vi "Create Error Cluster Control.vi"(5 "Error Cluster Sink":refnum<vi>, 6 "relative position/next to refnum":T1, 8 "error in (no error)":errorcluster, 10 "Indicator ?":bool, 11 "Diagram":refnum<vi>) -> (0 "error out":errorcluster, 2 "Terminal":refnum<vi>, 3 "cluster ref":refnum<vi>)   [LabVIEW 2012, in "Scripting Tools.lvlib"]
uses:
  Scripting Tools.lvlib
  <vilib>/Utility/miscctls.llb/LVPointTypeDef.ctl
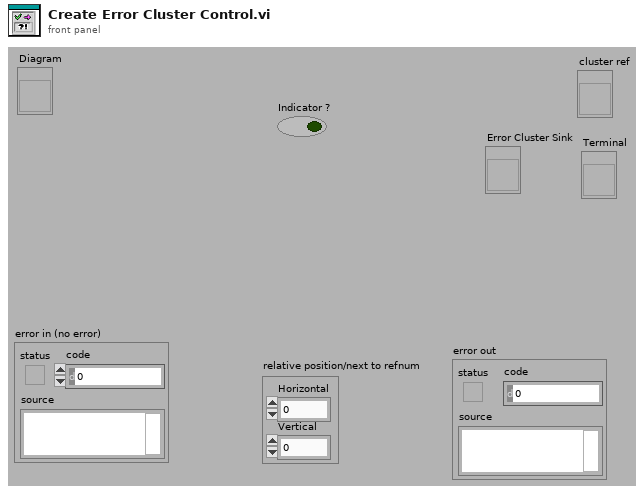
[diagram p1: front panel]
types:
  T1 = typedef "LVPointTypeDef.ctl" = cluster{"Horizontal":i16, "Vertical":i16}
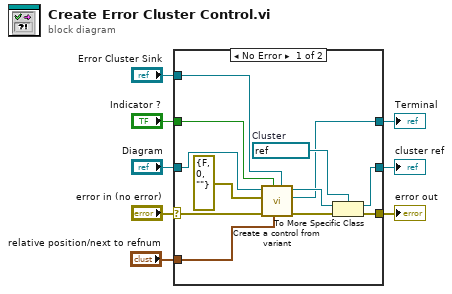
[diagram p0: block diagram]
diagram:
  n1 = case shown="No Error" "error in (no error)" {
    selector: "error in (no error)" -> [w20 w21]
    tunnel: "Indicator ?" -> [w17 _]
    tunnel: [w13 w21] -> w7
    tunnel: "relative position/next to refnum" -> [w19 _]
    tunnel: "Diagram" -> [w18 _]
    tunnel: "Error Cluster Sink" -> [w16 _]
    tunnel: [w10 _] -> w2
    tunnel: [w9 _] -> w1
    frame No Error {
      w11 = refnum<vi> refnum  # Cluster
      n2 = call <userlib>:"Create a control from variant.vi"("Terminal Source/Sink"=w16, "FP position"=w19, "Indicator?"=w17, "error in (no error)"=w20, "Constant Data"=errorcluster {"status"=FALSE, "code"=0, "source"=""} ("error IO"), "Diagram"=w18) -> ("error out"=w14:errorcluster, "Terminal"=w9:refnum<vi>, "Control Reference"=w12:refnum<vi>)  [unwired: 1 in, 2 out]
      n3 = To More Specific Class(target class=w11, reference=w12, error in=w14) -> (specific class reference=w10:refnum<vi>, error out=w13:errorcluster)
    }
    frame Error {
    }
  }
  "error out" <- w7
  "cluster ref" <- w2
  "Terminal" <- w1
